vi "Gen Fault Translation.vi"(3 "Gen Data":T1={"Alarms"=[], "Run Hours"=0.0, "Battery Voltage"=0.0, "Fuel Rate"=0.0, "Total Fuel"=0.0, "Power Factor"=0.0, "Active Power"=0.0, "Reactive Power"=0.0, "Apparent Power"=0.0, "Frequency"=0.0, "Status"=0, "Fault"=FALSE, "Alarm"=FALSE, "Com Fault"=TRUE, "Controller Mode"=0} {"Alarms" format="%04x"}) -> (1 "Gen Fault String":string)   [LabVIEW 2014]
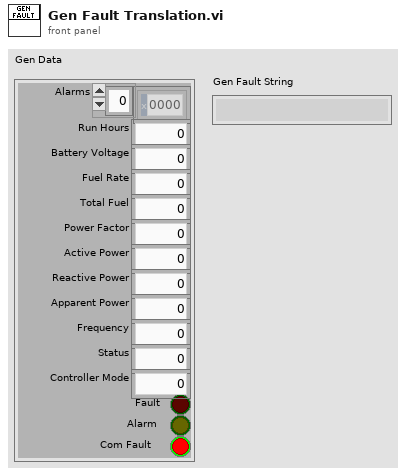
[diagram p1: front panel]
types:
  T1 = cluster{"Alarms":i16[], "Run Hours":dbl, "Battery Voltage":dbl, "Fuel Rate":dbl, "Total Fuel":dbl, "Power Factor":dbl, "Active Power":dbl, "Reactive Power":dbl, "Apparent Power":dbl, "Frequency":dbl, "Status":u16, "Fault":bool, "Alarm":bool, "Com Fault":bool, "Controller Mode":u16}
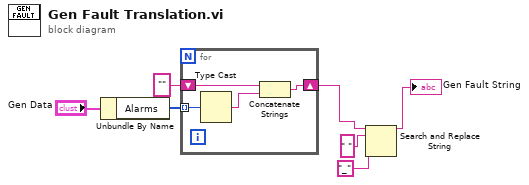
[diagram p0: block diagram]
diagram:
  n1 = Unbundle By Name("Gen Data") -> ("Alarms"=w5:i16[])
  n2 = for {
    tunnel: w5 -> [w11] mode=indexing
    shift-right: [w10] -> w2
    shift-left: "" -> [w8]
    n3 = Type Cast(x=w11) -> (*(type *) &x=w9:string)  [unwired: 1 in]
    n4 = Concatenate Strings(w8, w9) -> (w10:string)
  }
  n5 = Search and Replace String(input string=w2, search string=" ", replace string="_" ("replace string (\"\")")) -> (result string=→"Gen Fault String":string)  [unwired: 5 in, 3 out]
